vi "rsidr_core_global.vi"() -> ()   [LabVIEW 2015, in "Rohde&Schwarz CMXP NR FR2 Measurement.lvlib"] (continued)
{"Level"=5, "Class Only"=FALSE, "Identifier"="RSCMXPNRFR2M_ATTR_QUERY_MULTI_EVAL_MEASUREMENT_LIST_TERR_EXTREME_LIMIT_CHECK_RESULTS", "Descriptive Name"="Query Multi Eval Measurement List TERR Extreme Limit Check Results", "Data Type"=enum."RawString", "Command"="CALC:NRMM:MEAS{instance}:MEV:LIST:MOD:TERR:EXTR?", "Access"=enum."Read Only", "Range Table"="", "Read Callback"="", "Write Callback"="", "Range Callback"="", "Check Callback"="", "Rngtable Callback"="", "Coerce Callback"="", "Supported Models"="", "Instrument Options"="", "Check Status Callback"="", "Flags"=0, "Help"="Returns the limit check results for the transmit time error values for all measured list mode segments.\n\nAvailable Repeated Capabilities:\ninstance: i0, i1, i2, i3, i4, i5, i6, i7, i8, i9, i10, i11, i12, i13, i14, i15, i16, i17, i18, i19, i20, i21, i22, i23, i24, i25, i26, i27, i28, i29, i30, i31, i32\r\n\nRemote-control command(s):\nCALCulate:NRMMw:MEAS<i>:MEValuation:LIST:MODulation:TERRor:EXTReme?"}, {"Level"=5, "Class Only"=FALSE, "Identifier"="RSCMXPNRFR2M_ATTR_FETCH_MULTI_EVAL_MEASUREMENT_LIST_TERR_STANDARD_DEVIATION_RESULTS", "Descriptive Name"="Fetch Multi Eval Measurement List TERR Standard Deviation Results", "Data Type"=enum."RawString", "Command"="FETC:NRMM:MEAS{instance}:MEV:LIST:MOD:TERR:SDEV?", "Access"=enum."Read Only", "Range Table"="", "Read Callback"="", "Write Callback"="", "Range Callback"="", "Check Callback"="", "Rngtable Callback"="", "Coerce Callback"="", "Supported Models"="", "Instrument Options"="", "Check Status Callback"="", "Flags"=0, "Help"="Returns transmit time error values for all measured list mode segments.\n\nAvailable Repeated Capabilities:\ninstance: i0, i1, i2, i3, i4, i5, i6, i7, i8, i9, i10, i11, i12, i13, i14, i15, i16, i17, i18, i19, i20, i21, i22, i23, i24, i25, i26, i27, i28, i29, i30, i31, i32\r\n\nRemote-control command(s):\nFETCh:NRMMw:MEAS<i>:MEValuation:LIST:MODulation:TERRor:SDEViation?"}, {"Level"=4, "Class Only"=TRUE, "Identifier"="", "Descriptive Name"="User Equipment Power", "Data Type"=enum."ViInt32", "Command"="", "Access"=enum."Read Only", "Range Table"="", "Read Callback"="", "Write Callback"="", "Range Callback"="", "Check Callback"="", "Rngtable Callback"="", "Coerce Callback"="", "Supported Models"="", "Instrument Options"="", "Check Status Callback"="", "Flags"=0, "Help"="The following attributes return user equipment power values for all measured list mode segments."}, {"Level"=5, "Class Only"=FALSE, "Identifier"="RSCMXPNRFR2M_ATTR_FETCH_MULTI_EVAL_MEASUREMENT_LIST_TPOWER_AVERAGE_RESULTS", "Descriptive Name"="Fetch Multi Eval Measurement List TPower Average Results", "Data Type"=enum."RawString", "Command"="FETC:NRMM:MEAS{instance}:MEV:LIST:MOD:TPOW:AVER?", "Access"=enum."Read Only", "Range Table"="", "Read Callback"="", "Write Callback"="", "Range Callback"="", "Check Callback"="", "Rngtable Callback"="", "Coerce Callback"="", "Supported Models"="", "Instrument Options"="", "Check Status Callback"="", "Flags"=0, "Help"="Returns user equipment power values for all measured list mode segments.\n\nAvailable Repeated Capabilities:\ninstance: i0, i1, i2, i3, i4, i5, i6, i7, i8, i9, i10, i11, i12, i13, i14, i15, i16, i17, i18, i19, i20, i21, i22, i23, i24, i25, i26, i27, i28, i29, i30, i31, i32\r\n\nRemote-control command(s):\nFETCh:NRMMw:MEAS<i>:MEValuation:LIST:MODulation:TPOWer:AVERage?"}, {"Level"=5, "Class Only"=FALSE, "Identifier"="RSCMXPNRFR2M_ATTR_FETCH_MULTI_EVAL_MEASUREMENT_LIST_TPOWER_CURRENT_RESULTS", "Descriptive Name"="Fetch Multi Eval Measurement List TPower Current Results", "Data Type"=enum."RawString", "Command"="FETC:NRMM:MEAS{instance}:MEV:LIST:MOD:TPOW:CURR?", "Access"=enum."Read Only", "Range Table"="", "Read Callback"="", "Write Callback"="", "Range Callback"="", "Check Callback"="", "Rngtable Callback"="", "Coerce Callback"="", "Supported Models"="", "Instrument Options"="", "Check Status Callback"="", "Flags"=0, "Help"="Returns user equipment power values for all measured list mode segments.\n\nAvailable Repeated Capabilities:\ninstance: i0, i1, i2, i3, i4, i5, i6, i7, i8, i9, i10, i11, i12, i13, i14, i15, i16, i17, i18, i19, i20, i21, i22, i23, i24, i25, i26, i27, i28, i29, i30, i31, i32\r\n\nRemote-control command(s):\nFETCh:NRMMw:MEAS<i>:MEValuation:LIST:MODulation:TPOWer:CURRent?"}, {"Level"=5, "Class Only"=FALSE, "Identifier"="RSCMXPNRFR2M_ATTR_FETCH_MULTI_EVAL_MEASUREMENT_LIST_TPOWER_MAXIMUM_RESULTS", "Descriptive Name"="Fetch Multi Eval Measurement List TPower Maximum Results", "Data Type"=enum."RawString", "Command"="FETC:NRMM:MEAS{instance}:MEV:LIST:MOD:TPOW:MAX?", "Access"=enum."Read Only", "Range Table"="", "Read Callback"="", "Write Callback"="", "Range Callback"="", "Check Callback"="", "Rngtable Callback"="", "Coerce Callback"="", "Supported Models"="", "Instrument Options"="", "Check Status Callback"="", "Flags"=0, "Help"="Returns user equipment power values for all measured list mode segments.\n\nAvailable Repeated Capabilities:\ninstance: i0, i1, i2, i3, i4, i5, i6, i7, i8, i9, i10, i11, i12, i13, i14, i15, i16, i17, i18, i19, i20, i21, i22, i23, i24, i25, i26, i27, i28, i29, i30, i31, i32\r\n\nRemote-control command(s):\nFETCh:NRMMw:MEAS<i>:MEValuation:LIST:MODulation:TPOWer:MAXimum?"}, {"Level"=5, "Class Only"=FALSE, "Identifier"="RSCMXPNRFR2M_ATTR_FETCH_MULTI_EVAL_MEASUREMENT_LIST_TPOWER_MINIMUM_RESULTS", "Descriptive Name"="Fetch Multi Eval Measurement List TPower Minimum Results", "Data Type"=enum."RawString", "Command"="FETC:NRMM:MEAS{instance}:MEV:LIST:MOD:TPOW:MIN?", "Access"=enum."Read Only", "Range Table"="", "Read Callback"="", "Write Callback"="", "Range Callback"="", "Check Callback"="", "Rngtable Callback"="", "Coerce Callback"="", "Supported Models"="", "Instrument Options"="", "Check Status Callback"="", "Flags"=0, "Help"="Returns user equipment power values for all measured list mode segments.\n\nAvailable Repeated Capabilities:\ninstance: i0, i1, i2, i3, i4, i5, i6, i7, i8, i9, i10, i11, i12, i13, i14, i15, i16, i17, i18, i19, i20, i21, i22, i23, i24, i25, i26, i27, i28, i29, i30, i31, i32\r\n\nRemote-control command(s):\nFETCh:NRMMw:MEAS<i>:MEValuation:LIST:MODulation:TPOWer:MINimum?"}, {"Level"=5, "Class Only"=FALSE, "Identifier"="RSCMXPNRFR2M_ATTR_FETCH_MULTI_EVAL_MEASUREMENT_LIST_TPOWER_STANDARD_DEVIATION_RESULTS", "Descriptive Name"="Fetch Multi Eval Measurement List TPower Standard Deviation Results", "Data Type"=enum."RawString", "Command"="FETC:NRMM:MEAS{instance}:MEV:LIST:MOD:TPOW:SDEV?", "Access"=enum."Read Only", "Range Table"="", "Read Callback"="", "Write Callback"="", "Range Callback"="", "Check Callback"="", "Rngtable Callback"="", "Coerce Callback"="", "Supported Models"="", "Instrument Options"="", "Check Status Callback"="", "Flags"=0, "Help"="Returns user equipment power values for all measured list mode segments.\n\nAvailable Repeated Capabilities:\ninstance: i0, i1, i2, i3, i4, i5, i6, i7, i8, i9, i10, i11, i12, i13, i14, i15, i16, i17, i18, i19, i20, i21, i22, i23, i24, i25, i26, i27, i28, i29, i30, i31, i32\r\n\nRemote-control command(s):\nFETCh:NRMMw:MEAS<i>:MEValuation:LIST:MODulation:TPOWer:SDEViation?"}, {"Level"=5, "Class Only"=FALSE, "Identifier"="RSCMXPNRFR2M_ATTR_QUERY_MULTI_EVAL_MEASUREMENT_LIST_TPOWER_AVERAGE_LIMIT_CHECK_RESULTS", "Descriptive Name"="Query Multi Eval Measurement List TPower Average Limit Check Results", "Data Type"=enum."RawString", "Command"="CALC:NRMM:MEAS{instance}:MEV:LIST:MOD:TPOW:AVER?", "Access"=enum."Read Only", "Range Table"="", "Read Callback"="", "Write Callback"="", "Range Callback"="", "Check Callback"="", "Rngtable Callback"="", "Coerce Callback"="", "Supported Models"="", "Instrument Options"="", "Check Status Callback"="", "Flags"=0, "Help"="Returns the limit check results for the user equipment power values for all measured list mode segments.\n\nAvailable Repeated Capabilities:\ninstance: i0, i1, i2, i3, i4, i5, i6, i7, i8, i9, i10, i11, i12, i13, i14, i15, i16, i17, i18, i19, i20, i21, i22, i23, i24, i25, i26, i27, i28, i29, i30, i31, i32\r\n\nRemote-control command(s):\nCALCulate:NRMMw:MEAS<i>:MEValuation:LIST:MODulation:TPOWer:AVERage?"}, {"Level"=5, "Class Only"=FALSE, "Identifier"="RSCMXPNRFR2M_ATTR_QUERY_MULTI_EVAL_MEASUREMENT_LIST_TPOWER_CURRENT_LIMIT_CHECK_RESULTS", "Descriptive Name"="Query Multi Eval Measurement List TPower Current Limit Check Results", "Data Type"=enum."RawString", "Command"="CALC:NRMM:MEAS{instance}:MEV:LIST:MOD:TPOW:CURR?", "Access"=enum."Read Only", "Range Table"="", "Read Callback"="", "Write Callback"="", "Range Callback"="", "Check Callback"="", "Rngtable Callback"="", "Coerce Callback"="", "Supported Models"="", "Instrument Options"="", "Check Status Callback"="", "Flags"=0, "Help"="Returns the limit check results for the user equipment power values for all measured list mode segments.\n\nAvailable Repeated Capabilities:\ninstance: i0, i1, i2, i3, i4, i5, i6, i7, i8, i9, i10, i11, i12, i13, i14, i15, i16, i17, i18, i19, i20, i21, i22, i23, i24, i25, i26, i27, i28, i29, i30, i31, i32\r\n\nRemote-control command(s):\nCALCulate:NRMMw:MEAS<i>:MEValuation:LIST:MODulation:TPOWer:CURRent?"}, {"Level"=5, "Class Only"=FALSE, "Identifier"="RSCMXPNRFR2M_ATTR_QUERY_MULTI_EVAL_MEASUREMENT_LIST_TPOWER_MAXIMUM_LIMIT_CHECK_RESULTS", "Descriptive Name"="Query Multi Eval Measurement List TPower Maximum Limit Check Results", "Data Type"=enum."RawString", "Command"="CALC:NRMM:MEAS{instance}:MEV:LIST:MOD:TPOW:MAX?", "Access"=enum."Read Only", "Range Table"="", "Read Callback"="", "Write Callback"="", "Range Callback"="", "Check Callback"="", "Rngtable Callback"="", "Coerce Callback"="", "Supported Models"="", "Instrument Options"="", "Check Status Callback"="", "Flags"=0, "Help"="Returns the limit check results for the user equipment power values for all measured list mode segments.\n\nAvailable Repeated Capabilities:\ninstance: i0, i1, i2, i3, i4, i5, i6, i7, i8, i9, i10, i11, i12, i13, i14, i15, i16, i17, i18, i19, i20, i21, i22, i23, i24, i25, i26, i27, i28, i29, i30, i31, i32\r\n\nRemote-control command(s):\nCALCulate:NRMMw:MEAS<i>:MEValuation:LIST:MODulation:TPOWer:MAXimum?"}, {"Level"=5, "Class Only"=FALSE, "Identifier"="RSCMXPNRFR2M_ATTR_QUERY_MULTI_EVAL_MEASUREMENT_LIST_TPOWER_MINIMUM_LIMIT_CHECK_RESULTS", "Descriptive Name"="Query Multi Eval Measurement List TPower Minimum Limit Check Results", "Data Type"=enum."RawString", "Command"="CALC:NRMM:MEAS{instance}:MEV:LIST:MOD:TPOW:MIN?", "Access"=enum."Read Only", "Range Table"="", "Read Callback"="", "Write Callback"="", "Range Callback"="", "Check Callback"="", "Rngtable Callback"="", "Coerce Callback"="", "Supported Models"="", "Instrument Options"="", "Check Status Callback"="", "Flags"=0, "Help"="Returns the limit check results for the user equipment power values for all measured list mode segments.\n\nAvailable Repeated Capabilities:\ninstance: i0, i1, i2, i3, i4, i5, i6, i7, i8, i9, i10, i11, i12, i13, i14, i15, i16, i17, i18, i19, i20, i21, i22, i23, i24, i25, i26, i27, i28, i29, i30, i31, i32\r\n\nRemote-control command(s):\nCALCulate:NRMMw:MEAS<i>:MEValuation:LIST:MODulation:TPOWer:MINimum?"}, {"Level"=4, "Class Only"=TRUE, "Identifier"="", "Descriptive Name"="Modulation", "Data Type"=enum."ViInt32", "Command"="", "Access"=enum."Read Only", "Range Table"="", "Read Callback"="", "Write Callback"="", "Range Callback"="", "Check Callback"="", "Rngtable Callback"="", "Coerce Callback"="", "Supported Models"="", "Instrument Options"="", "Check Status Callback"="", "Flags"=0, "Help"="The following attributes return the detected modulation scheme for all measured list mode segments."}, {"Level"=5, "Class Only"=FALSE, "Identifier"="RSCMXPNRFR2M_ATTR_FETCH_MULTI_EVAL_MEASUREMENT_LIST_MODULATION_DETECTED_ALLOCATION_RESULTS", "Descriptive Name"="Fetch Multi Eval Measurement List Modulation Detected Allocation Results", "Data Type"=enum."RawString", "Command"="FETC:NRMM:MEAS{instance}:MEV:LIST:MOD:DALL?", "Access"=enum."Read Only", "Range Table"="", "Read Callback"="", "Write Callback"="", "Range Callback"="", "Check Callback"="", "Rngtable Callback"="", "Coerce Callback"="", "Supported Models"="", "Instrument Options"="", "Check Status Callback"="", "Flags"=0, "Help"="Returns the detected allocation for all measured list mode segments.\n\nAvailable Repeated Capabilities:\ninstance: i0, i1, i2, i3, i4, i5, i6, i7, i8, i9, i10, i11, i12, i13, i14, i15, i16, i17, i18, i19, i20, i21, i22, i23, i24, i25, i26, i27, i28, i29, i30, i31, i32\r\n\nRemote-control command(s):\nFETCh:NRMMw:MEAS<i>:MEValuation:LIST:MODulation:DALLocation?"}, {"Level"=5, "Class Only"=FALSE, "Identifier"="RSCMXPNRFR2M_ATTR_FETCH_MULTI_EVAL_MEASUREMENT_LIST_MODULATION_DETECTED_MODULATION_RESULTS", "Descriptive Name"="Fetch Multi Eval Measurement List Modulation Detected Modulation Results", "Data Type"=enum."RawString", "Command"="FETC:NRMM:MEAS{instance}:MEV:LIST:MOD:DMOD?", "Access"=enum."Read Only", "Range Table"="", "Read Callback"="", "Write Callback"="", "Range Callback"="", "Check Callback"="", "Rngtable Callback"="", "Coerce Callback"="", "Supported Models"="", "Instrument Options"="", "Check Status Callback"="", "Flags"=0, "Help"="Returns the detected modulation scheme for all measured list mode segments.\n\nAvailable Repeated Capabilities:\ninstance: i0, i1, i2, i3, i4, i5, i6, i7, i8, i9, i10, i11, i12, i13, i14, i15, i16, i17, i18, i19, i20, i21, i22, i23, i24, i25, i26, i27, i28, i29, i30, i31, i32\r\n\nRemote-control command(s):\nFETCh:NRMMw:MEAS<i>:MEValuation:LIST:MODulation:DMODulation?"}, {"Level"=4, "Class Only"=TRUE, "Identifier"="", "Descriptive Name"="Spectrum Emission Mask", "Data Type"=enum."ViInt32", "Command"="", "Access"=enum."Read Only", "Range Table"="", "Read Callback"="", "Write Callback"="", "Range Callback"="", "Check Callback"="", "Rngtable Callback"="", "Coerce Callback"="", "Supported Models"="", "Instrument Options"="", "Check Status Callback"="", "Flags"=0, "Help"="The following attributes return the occupied bandwidth for all measured list mode segments."}, {"Level"=5, "Class Only"=FALSE, "Identifier"="RSCMXPNRFR2M_ATTR_FETCH_MULTI_EVAL_MEASUREMENT_LIST_SEM_OBW_AVERAGE_RESULTS", "Descriptive Name"="Fetch Multi Eval Measurement List SEM OBW Average Results", "Data Type"=enum."RawString", "Command"="FETC:NRMM:MEAS{instance}:MEV:LIST:SEM:OBW:AVER?", "Access"=enum."Read Only", "Range Table"="", "Read Callback"="", "Write Callback"="", "Range Callback"="", "Check Callback"="", "Rngtable Callback"="", "Coerce Callback"="", "Supported Models"="", "Instrument Options"="", "Check Status Callback"="", "Flags"=0, "Help"="Returns the occupied bandwidth for all measured list mode segments.\n\nAvailable Repeated Capabilities:\ninstance: i0, i1, i2, i3, i4, i5, i6, i7, i8, i9, i10, i11, i12, i13, i14, i15, i16, i17, i18, i19, i20, i21, i22, i23, i24, i25, i26, i27, i28, i29, i30, i31, i32\r\n\nRemote-control command(s):\nFETCh:NRMMw:MEAS<i>:MEValuation:LIST:SEMask:OBW:AVERage?"}, {"Level"=5, "Class Only"=FALSE, "Identifier"="RSCMXPNRFR2M_ATTR_FETCH_MULTI_EVAL_MEASUREMENT_LIST_SEM_OBW_CURRENT_RESULTS", "Descriptive Name"="Fetch Multi Eval Measurement List SEM OBW Current Results", "Data Type"=enum."RawString", "Command"="FETC:NRMM:MEAS{instance}:MEV:LIST:SEM:OBW:CURR?", "Access"=enum."Read Only", "Range Table"="", "Read Callback"="", "Write Callback"="", "Range Callback"="", "Check Callback"="", "Rngtable Callback"="", "Coerce Callback"="", "Supported Models"="", "Instrument Options"="", "Check Status Callback"="", "Flags"=0, "Help"="Returns the occupied bandwidth for all measured list mode segments.\n\nAvailable Repeated Capabilities:\ninstance: i0, i1, i2, i3, i4, i5, i6, i7, i8, i9, i10, i11, i12, i13, i14, i15, i16, i17, i18, i19, i20, i21, i22, i23, i24, i25, i26, i27, i28, i29, i30, i31, i32\r\n\nRemote-control command(s):\nFETCh:NRMMw:MEAS<i>:MEValuation:LIST:SEMask:OBW:CURRent?"}, {"Level"=5, "Class Only"=FALSE, "Identifier"="RSCMXPNRFR2M_ATTR_FETCH_MULTI_EVAL_MEASUREMENT_LIST_SEM_OBW_EXTREME_RESULTS", "Descriptive Name"="Fetch Multi Eval Measurement List SEM OBW Extreme Results", "Data Type"=enum."RawString", "Command"="FETC:NRMM:MEAS{instance}:MEV:LIST:SEM:OBW:EXTR?", "Access"=enum."Read Only", "Range Table"="", "Read Callback"="", "Write Callback"="", "Range Callback"="", "Check Callback"="", "Rngtable Callback"="", "Coerce Callback"="", "Supported Models"="", "Instrument Options"="", "Check Status Callback"="", "Flags"=0, "Help"="Returns the occupied bandwidth for all measured list mode segments.\n\nAvailable Repeated Capabilities:\ninstance: i0, i1, i2, i3, i4, i5, i6, i7, i8, i9, i10, i11, i12, i13, i14, i15, i16, i17, i18, i19, i20, i21, i22, i23, i24, i25, i26, i27, i28, i29, i30, i31, i32\r\n\nRemote-control command(s):\nFETCh:NRMMw:MEAS<i>:MEValuation:LIST:SEMask:OBW:EXTReme?"}, {"Level"=5, "Class Only"=FALSE, "Identifier"="RSCMXPNRFR2M_ATTR_FETCH_MULTI_EVAL_MEASUREMENT_LIST_SEM_OBW_STANDARD_DEVIATION_RESULTS", "Descriptive Name"="Fetch Multi Eval Measurement List SEM OBW Standard Deviation Results", "Data Type"=enum."RawString", "Command"="FETC:NRMM:MEAS{instance}:MEV:LIST:SEM:OBW:SDEV?", "Access"=enum."Read Only", "Range Table"="", "Read Callback"="", "Write Callback"="", "Range Callback"="", "Check Callback"="", "Rngtable Callback"="", "Coerce Callback"="", "Supported Models"="", "Instrument Options"="", "Check Status Callback"="", "Flags"=0, "Help"="Returns the occupied bandwidth for all measured list mode segments.\n\nAvailable Repeated Capabilities:\ninstance: i0, i1, i2, i3, i4, i5, i6, i7, i8, i9, i10, i11, i12, i13, i14, i15, i16, i17, i18, i19, i20, i21, i22, i23, i24, i25, i26, i27, i28, i29, i30, i31, i32\r\n\nRemote-control command(s):\nFETCh:NRMMw:MEAS<i>:MEValuation:LIST:SEMask:OBW:SDEViation?"}, {"Level"=5, "Class Only"=FALSE, "Identifier"="RSCMXPNRFR2M_ATTR_QUERY_MULTI_EVAL_MEASUREMENT_LIST_SEM_OBW_AVERAGE_LIMIT_CHECK_RESULTS", "Descriptive Name"="Query Multi Eval Measurement List SEM OBW Average Limit Check Results", "Data Type"=enum."RawString", "Command"="CALC:NRMM:MEAS{instance}:MEV:LIST:SEM:OBW:AVER?", "Access"=enum."Read Only", "Range Table"="", "Read Callback"="", "Write Callback"="", "Range Callback"="", "Check Callback"="", "Rngtable Callback"="", "Coerce Callback"="", "Supported Models"="", "Instrument Options"="", "Check Status Callback"="", "Flags"=0, "Help"="Returns the limit check results for the occupied bandwidth for all measured list mode segments.\n\nAvailable Repeated Capabilities:\ninstance: i0, i1, i2, i3, i4, i5, i6, i7, i8, i9, i10, i11, i12, i13, i14, i15, i16, i17, i18, i19, i20, i21, i22, i23, i24, i25, i26, i27, i28, i29, i30, i31, i32\r\n\nRemote-control command(s):\nCALCulate:NRMMw:MEAS<i>:MEValuation:LIST:SEMask:OBW:AVERage?"}, {"Level"=5, "Class Only"=FALSE, "Identifier"="RSCMXPNRFR2M_ATTR_QUERY_MULTI_EVAL_MEASUREMENT_LIST_SEM_OBW_CURRENT_LIMIT_CHECK_RESULTS", "Descriptive Name"="Query Multi Eval Measurement List SEM OBW Current Limit Check Results", "Data Type"=enum."RawString", "Command"="CALC:NRMM:MEAS{instance}:MEV:LIST:SEM:OBW:CURR?", "Access"=enum."Read Only", "Range Table"="", "Read Callback"="", "Write Callback"="", "Range Callback"="", "Check Callback"="", "Rngtable Callback"="", "Coerce Callback"="", "Supported Models"="", "Instrument Options"="", "Check Status Callback"="", "Flags"=0, "Help"="Returns the limit check results for the occupied bandwidth for all measured list mode segments.\n\nAvailable Repeated Capabilities:\ninstance: i0, i1, i2, i3, i4, i5, i6, i7, i8, i9, i10, i11, i12, i13, i14, i15, i16, i17, i18, i19, i20, i21, i22, i23, i24, i25, i26, i27, i28, i29, i30, i31, i32\r\n\nRemote-control command(s):\nCALCulate:NRMMw:MEAS<i>:MEValuation:LIST:SEMask:OBW:CURRent?"}, {"Level"=5, "Class Only"=FALSE, "Identifier"="RSCMXPNRFR2M_ATTR_QUERY_MULTI_EVAL_MEASUREMENT_LIST_SEM_OBW_EXTREME_LIMIT_CHECK_RESULTS", "Descriptive Name"="Query Multi Eval Measurement List SEM OBW Extreme Limit Check Results", "Data Type"=enum."RawString", "Command"="CALC:NRMM:MEAS{instance}:MEV:LIST:SEM:OBW:EXTR?", "Access"=enum."Read Only", "Range Table"="", "Read Callback"="", "Write Callback"="", "Range Callback"="", "Check Callback"="", "Rngtable Callback"="", "Coerce Callback"="", "Supported Models"="", "Instrument Options"="", "Check Status Callback"="", "Flags"=0, "Help"="Returns the limit check results for the occupied bandwidth for all measured list mode segments.\n\nAvailable Repeated Capabilities:\ninstance: i0, i1, i2, i3, i4, i5, i6, i7, i8, i9, i10, i11, i12, i13, i14, i15, i16, i17, i18, i19, i20, i21, i22, i23, i24, i25, i26, i27, i28, i29, i30, i31, i32\r\n\nRemote-control command(s):\nCALCulate:NRMMw:MEAS<i>:MEValuation:LIST:SEMask:OBW:EXTReme?"}, {"Level"=5, "Class Only"=FALSE, "Identifier"="RSCMXPNRFR2M_ATTR_FETCH_MULTI_EVAL_MEASUREMENT_LIST_SEM_TX_POWER_AVERAGE_RESULTS", "Descriptive Name"="Fetch Multi Eval Measurement List SEM TX Power Average Results", "Data Type"=enum."RawString", "Command"="FETC:NRMM:MEAS{instance}:MEV:LIST:SEM:TXP:AVER?", "Access"=enum."Read Only", "Range Table"="", "Read Callback"="", "Write Callback"="", "Range Callback"="", "Check Callback"="", "Rngtable Callback"="", "Coerce Callback"="", "Supported Models"="", "Instrument Options"="", "Check Status Callback"="", "Flags"=0, "Help"="Returns the total TX power in the slot for all measured list mode segments.\n\nAvailable Repeated Capabilities:\ninstance: i0, i1, i2, i3, i4, i5, i6, i7, i8, i9, i10, i11, i12, i13, i14, i15, i16, i17, i18, i19, i20, i21, i22, i23, i24, i25, i26, i27, i28, i29, i30, i31, i32\r\n\nRemote-control command(s):\nFETCh:NRMMw:MEAS<i>:MEValuation:LIST:SEMask:TXPower:AVERage?"}, {"Level"=5, "Class Only"=FALSE, "Identifier"="RSCMXPNRFR2M_ATTR_FETCH_MULTI_EVAL_MEASUREMENT_LIST_SEM_TX_POWER_CURRENT_RESULTS", "Descriptive Name"="Fetch Multi Eval Measurement List SEM TX Power Current Results", "Data Type"=enum."RawString", "Command"="FETC:NRMM:MEAS{instance}:MEV:LIST:SEM:TXP:CURR?", "Access"=enum."Read Only", "Range Table"="", "Read Callback"="", "Write Callback"="", "Range Callback"="", "Check Callback"="", "Rngtable Callback"="", "Coerce Callback"="", "Supported Models"="", "Instrument Options"="", "Check Status Callback"="", "Flags"=0, "Help"="Returns the total TX power in the slot for all measured list mode segments.\n\nAvailable Repeated Capabilities:\ninstance: i0, i1, i2, i3, i4, i5, i6, i7, i8, i9, i10, i11, i12, i13, i14, i15, i16, i17, i18, i19, i20, i21, i22, i23, i24, i25, i26, i27, i28, i29, i30, i31, i32\r\n\nRemote-control command(s):\nFETCh:NRMMw:MEAS<i>:MEValuation:LIST:SEMask:TXPower:CURRent?"}, {"Level"=5, "Class Only"=FALSE, "Identifier"="RSCMXPNRFR2M_ATTR_FETCH_MULTI_EVAL_MEASUREMENT_LIST_SEM_TX_POWER_STANDARD_DEVIATION_RESULTS", "Descriptive Name"="Fetch Multi Eval Measurement List SEM TX Power Standard Deviation Results", "Data Type"=enum."RawString", "Command"="FETC:NRMM:MEAS{instance}:MEV:LIST:SEM:TXP:SDEV?", "Access"=enum."Read Only", "Range Table"="", "Read Callback"="", "Write Callback"="", "Range Callback"="", "Check Callback"="", "Rngtable Callback"="", "Coerce Callback"="", "Supported Models"="", "Instrument Options"="", "Check Status Callback"="", "Flags"=0, "Help"="Returns the total TX power in the slot for all measured list mode segments.\n\nAvailable Repeated Capabilities:\ninstance: i0, i1, i2, i3, i4, i5, i6, i7, i8, i9, i10, i11, i12, i13, i14, i15, i16, i17, i18, i19, i20, i21, i22, i23, i24, i25, i26, i27, i28, i29, i30, i31, i32\r\n\nRemote-control command(s):\nFETCh:NRMMw:MEAS<i>:MEValuation:LIST:SEMask:TXPower:SDEViation?"}, {"Level"=5, "Class Only"=FALSE, "Identifier"="RSCMXPNRFR2M_ATTR_FETCH_MULTI_EVAL_MEASUREMENT_LIST_SEM_TX_POWER_MAXIMUM_RESULTS", "Descriptive Name"="Fetch Multi Eval Measurement List SEM TX Power Maximum Results", "Data Type"=enum."RawString", "Command"="FETC:NRMM:MEAS{instance}:MEV:LIST:SEM:TXP:MAX?", "Access"=enum."Read Only", "Range Table"="", "Read Callback"="", "Write Callback"="", "Range Callback"="", "Check Callback"="", "Rngtable Callback"="", "Coerce Callback"="", "Supported Models"="", "Instrument Options"="", "Check Status Callback"="", "Flags"=0, "Help"="Returns the total TX power in the slot for all measured list mode segments.\n\nAvailable Repeated Capabilities:\ninstance: i0, i1, i2, i3, i4, i5, i6, i7, i8, i9, i10, i11, i12, i13, i14, i15, i16, i17, i18, i19, i20, i21, i22, i23, i24, i25, i26, i27, i28, i29, i30, i31, i32\r\n\nRemote-control command(s):\nFETCh:NRMMw:MEAS<i>:MEValuation:LIST:SEMask:TXPower:MAXimum?"}, {"Level"=5, "Class Only"=FALSE, "Identifier"="RSCMXPNRFR2M_ATTR_FETCH_MULTI_EVAL_MEASUREMENT_LIST_SEM_TX_POWER_MINIMUM_RESULTS", "Descriptive Name"="Fetch Multi Eval Measurement List SEM TX Power Minimum Results", "Data Type"=enum."RawString", "Command"="FETC:NRMM:MEAS{instance}:MEV:LIST:SEM:TXP:MIN?", "Access"=enum."Read Only", "Range Table"="", "Read Callback"="", "Write Callback"="", "Range Callback"="", "Check Callback"="", "Rngtable Callback"="", "Coerce Callback"="", "Supported Models"="", "Instrument Options"="", "Check Status Callback"="", "Flags"=0, "Help"="Returns the total TX power in the slot for all measured list mode segments.\n\nAvailable Repeated Capabilities:\ninstance: i0, i1, i2, i3, i4, i5, i6, i7, i8, i9, i10, i11, i12, i13, i14, i15, i16, i17, i18, i19, i20, i21, i22, i23, i24, i25, i26, i27, i28, i29, i30, i31, i32\r\n\nRemote-control command(s):\nFETCh:NRMMw:MEAS<i>:MEValuation:LIST:SEMask:TXPower:MINimum?"}, {"Level"=5, "Class Only"=FALSE, "Identifier"="RSCMXPNRFR2M_ATTR_QUERY_MULTI_EVAL_MEASUREMENT_LIST_SEM_TX_POWER_AVERAGE_LIMIT_CHECK_RESULTS", "Descriptive Name"="Query Multi Eval Measurement List SEM TX Power Average Limit Check Results", "Data Type"=enum."RawString", "Command"="CALC:NRMM:MEAS{instance}:MEV:LIST:SEM:TXP:AVER?", "Access"=enum."Read Only", "Range Table"="", "Read Callback"="", "Write Callback"="", "Range Callback"="", "Check Callback"="", "Rngtable Callback"="", "Coerce Callback"="", "Supported Models"="", "Instrument Options"="", "Check Status Callback"="", "Flags"=0, "Help"="Returns the limit check results for the total TX power in the slot for all measured list mode segments.\n\nAvailable Repeated Capabilities:\ninstance: i0, i1, i2, i3, i4, i5, i6, i7, i8, i9, i10, i11, i12, i13, i14, i15, i16, i17, i18, i19, i20, i21, i22, i23, i24, i25, i26, i27, i28, i29, i30, i31, i32\r\n\nRemote-control command(s):\nCALCulate:NRMMw:MEAS<i>:MEValuation:LIST:SEMask:TXPower:AVERage?"}, {"Level"=5, "Class Only"=FALSE, "Identifier"="RSCMXPNRFR2M_ATTR_QUERY_MULTI_EVAL_MEASUREMENT_LIST_SEM_TX_POWER_CURRENT_LIMIT_CHECK_RESULTS", "Descriptive Name"="Query Multi Eval Measurement List SEM TX Power Current Limit Check Results", "Data Type"=enum."RawString", "Command"="CALC:NRMM:MEAS{instance}:MEV:LIST:SEM:TXP:CURR?", "Access"=enum."Read Only", "Range Table"="", "Read Callback"="", "Write Callback"="", "Range Callback"="", "Check Callback"="", "Rngtable Callback"="", "Coerce Callback"="", "Supported Models"="", "Instrument Options"="", "Check Status Callback"="", "Flags"=0, "Help"="Returns the limit check results for the total TX power in the slot for all measured list mode segments.\n\nAvailable Repeated Capabilities:\ninstance: i0, i1, i2, i3, i4, i5, i6, i7, i8, i9, i10, i11, i12, i13, i14, i15, i16, i17, i18, i19, i20, i21, i22, i23, i24, i25, i26, i27, i28, i29, i30, i31, i32\r\n\nRemote-control command(s):\nCALCulate:NRMMw:MEAS<i>:MEValuation:LIST:SEMask:TXPower:CURRent?"}, {"Level"=5, "Class Only"=FALSE, "Identifier"="RSCMXPNRFR2M_ATTR_QUERY_MULTI_EVAL_MEASUREMENT_LIST_SEM_TX_POWER_MAXIMUM_LIMIT_CHECK_RESULTS", "Descriptive Name"="Query Multi Eval Measurement List SEM TX Power Maximum Limit Check Results", "Data Type"=enum."RawString", "Command"="CALC:NRMM:MEAS{instance}:MEV:LIST:SEM:TXP:MAX?", "Access"=enum."Read Only", "Range Table"="", "Read Callback"="", "Write Callback"="", "Range Callback"="", "Check Callback"="", "Rngtable Callback"="", "Coerce Callback"="", "Supported Models"="", "Instrument Options"="", "Check Status Callback"="", "Flags"=0, "Help"="Returns the limit check results for the total TX power in the slot for all measured list mode segments.\n\nAvailable Repeated Capabilities:\ninstance: i0, i1, i2, i3, i4, i5, i6, i7, i8, i9, i10, i11, i12, i13, i14, i15, i16, i17, i18, i19, i20, i21, i22, i23, i24, i25, i26, i27, i28, i29, i30, i31, i32\r\n\nRemote-control command(s):\nCALCulate:NRMMw:MEAS<i>:MEValuation:LIST:SEMask:TXPower:MAXimum?"}, {"Level"=5, "Class Only"=FALSE, "Identifier"="RSCMXPNRFR2M_ATTR_QUERY_MULTI_EVAL_MEASUREMENT_LIST_SEM_TX_POWER_MINIMUM_LIMIT_CHECK_RESULTS", "Descriptive Name"="Query Multi Eval Measurement List SEM TX Power Minimum Limit Check Results", "Data Type"=enum."RawString", "Command"="CALC:NRMM:MEAS{instance}:MEV:LIST:SEM:TXP:MIN?", "Access"=enum."Read Only", "Range Table"="", "Read Callback"="", "Write Callback"="", "Range Callback"="", "Check Callback"="", "Rngtable Callback"="", "Coerce Callback"="", "Supported Models"="", "Instrument Options"="", "Check Status Callback"="", "Flags"=0, "Help"="Returns the limit check results for the total TX power in the slot for all measured list mode segments.\n\nAvailable Repeated Capabilities:\ninstance: i0, i1, i2, i3, i4, i5, i6, i7, i8, i9, i10, i11, i12, i13, i14, i15, i16, i17, i18, i19, i20, i21, i22, i23, i24, i25, i26, i27, i28, i29, i30, i31, i32\r\n\nRemote-control command(s):\nCALCulate:NRMMw:MEAS<i>:MEValuation:LIST:SEMask:TXPower:MINimum?"}, {"Level"=5, "Class Only"=FALSE, "Identifier"="RSCMXPNRFR2M_ATTR_FETCH_MULTI_EVAL_MEASUREMENT_LIST_SEM_DETECTED_ALLOCATION_RESULTS", "Descriptive Name"="Fetch Multi Eval Measurement List SEM Detected Allocation Results", "Data Type"=enum."RawString", "Command"="FETC:NRMM:MEAS{instance}:MEV:LIST:SEM:DALL?", "Access"=enum."Read Only", "Range Table"="", "Read Callback"="", "Write Callback"="", "Range Callback"="", "Check Callback"="", "Rngtable Callback"="", "Coerce Callback"="", "Supported Models"="", "Instrument Options"="", "Check Status Callback"="", "Flags"=0, "Help"="Returns the detected allocation for all measured list mode segments.\n\nAvailable Repeated Capabilities:\ninstance: i0, i1, i2, i3, i4, i5, i6, i7, i8, i9, i10, i11, i12, i13, i14, i15, i16, i17, i18, i19, i20, i21, i22, i23, i24, i25, i26, i27, i28, i29, i30, i31, i32\r\n\nRemote-control command(s):\nFETCh:NRMMw:MEAS<i>:MEValuation:LIST:SEMask:DALLocation?"}, {"Level"=5, "Class Only"=TRUE, "Identifier"="", "Descriptive Name"="Area", "Data Type"=enum."ViInt32", "Command"="", "Access"=enum."Read Only", "Range Table"="", "Read Callback"="", "Write Callback"="", "Range Callback"="", "Check Callback"="", "Rngtable Callback"="", "Coerce Callback"="", "Supported Models"="", "Instrument Options"="", "Check Status Callback"="", "Flags"=0, "Help"="The following attributes return spectrum emission mask margin positions for all measured list mode segments."}, {"Level"=6, "Class Only"=FALSE, "Identifier"="RSCMXPNRFR2M_ATTR_FETCH_MULTI_EVAL_MEASUREMENT_LIST_SEM_MARGIN_AREA_NEGATIVE_AVERAGE_RESULTS", "Descriptive Name"="Fetch Multi Eval Measurement List SEM Margin Area Negative Average Results", "Data Type"=enum."RawString", "Command"="FETC:NRMM:MEAS{instance}:MEV:LIST:SEM:MARG:AREA{Area}:NEG:AVER?", "Access"=enum."Read Only", "Range Table"="", "Read Callback"="", "Write Callback"="", "Range Callback"="", "Check Callback"="", "Rngtable Callback"="", "Coerce Callback"="", "Supported Models"="", "Instrument Options"="", "Check Status Callback"="", "Flags"=0, "Help"="Returns spectrum emission mask margin positions for all measured list mode segments.\n\nAvailable Repeated Capabilities:\ninstance: i0, i1, i2, i3, i4, i5, i6, i7, i8, i9, i10, i11, i12, i13, i14, i15, i16, i17, i18, i19, i20, i21, i22, i23, i24, i25, i26, i27, i28, i29, i30, i31, i32\r\nArea: a1, a2, a3, a4, a5, a6, a7, a8, a9, a10, a11, a12\r\n\nRemote-control command(s):\nFETCh:NRMMw:MEAS<i>:MEValuation:LIST:SEMask:MARGin:AREA<no>:NEGativ:AVERage?"}, {"Level"=6, "Class Only"=FALSE, "Identifier"="RSCMXPNRFR2M_ATTR_FETCH_MULTI_EVAL_MEASUREMENT_LIST_SEM_MARGIN_AREA_NEGATIVE_CURRENT_RESULTS", "Descriptive Name"="Fetch Multi Eval Measurement List SEM Margin Area Negative Current Results", "Data Type"=enum."RawString", "Command"="FETC:NRMM:MEAS{instance}:MEV:LIST:SEM:MARG:AREA{Area}:NEG:CURR?", "Access"=enum."Read Only", "Range Table"="", "Read Callback"="", "Write Callback"="", "Range Callback"="", "Check Callback"="", "Rngtable Callback"="", "Coerce Callback"="", "Supported Models"="", "Instrument Options"="", "Check Status Callback"="", "Flags"=0, "Help"="Returns spectrum emission mask margin positions for all measured list mode segments.\n\nAvailable Repeated Capabilities:\ninstance: i0, i1, i2, i3, i4, i5, i6, i7, i8, i9, i10, i11, i12, i13, i14, i15, i16, i17, i18, i19, i20, i21, i22, i23, i24, i25, i26, i27, i28, i29, i30, i31, i32\r\nArea: a1, a2, a3, a4, a5, a6, a7, a8, a9, a10, a11, a12\r\n\nRemote-control command(s):\nFETCh:NRMMw:MEAS<i>:MEValuation:LIST:SEMask:MARGin:AREA<no>:NEGativ:CURRent?"}, {"Level"=6, "Class Only"=FALSE, "Identifier"="RSCMXPNRFR2M_ATTR_FETCH_MULTI_EVAL_MEASUREMENT_LIST_SEM_MARGIN_AREA_NEGATIVE_MINIMUM_RESULTS", "Descriptive Name"="Fetch Multi Eval Measurement List SEM Margin Area Negative Minimum Results", "Data Type"=enum."RawString", "Command"="FETC:NRMM:MEAS{instance}:MEV:LIST:SEM:MARG:AREA{Area}:NEG:MIN?", "Access"=enum."Read Only", "Range Table"="", "Read Callback"="", "Write Callback"="", "Range Callback"="", "Check Callback"="", "Rngtable Callback"="", "Coerce Callback"="", "Supported Models"="", "Instrument Options"="", "Check Status Callback"="", "Flags"=0, "Help"="Returns spectrum emission mask margin positions for all measured list mode segments.\n\nAvailable Repeated Capabilities:\ninstance: i0, i1, i2, i3, i4, i5, i6, i7, i8, i9, i10, i11, i12, i13, i14, i15, i16, i17, i18, i19, i20, i21, i22, i23, i24, i25, i26, i27, i28, i29, i30, i31, i32\r\nArea: a1, a2, a3, a4, a5, a6, a7, a8, a9, a10, a11, a12\r\n\nRemote-control command(s):\nFETCh:NRMMw:MEAS<i>:MEValuation:LIST:SEMask:MARGin:AREA<no>:NEGativ:MINimum?"}, {"Level"=6, "Class Only"=FALSE, "Identifier"="RSCMXPNRFR2M_ATTR_FETCH_MULTI_EVAL_MEASUREMENT_LIST_SEM_MARGIN_AREA_POSITIVE_AVERAGE_RESULTS", "Descriptive Name"="Fetch Multi Eval Measurement List SEM Margin Area Positive Average Results", "Data Type"=enum."RawString", "Command"="FETC:NRMM:MEAS{instance}:MEV:LIST:SEM:MARG:AREA{Area}:POS:AVER?", "Access"=enum."Read Only", "Range Table"="", "Read Callback"="", "Write Callback"="", "Range Callback"="", "Check Callback"="", "Rngtable Callback"="", "Coerce Callback"="", "Supported Models"="", "Instrument Options"="", "Check Status Callback"="", "Flags"=0, "Help"="Returns spectrum emission mask margin positions for all measured list mode segments.\n\nAvailable Repeated Capabilities:\ninstance: i0, i1, i2, i3, i4, i5, i6, i7, i8, i9, i10, i11, i12, i13, i14, i15, i16, i17, i18, i19, i20, i21, i22, i23, i24, i25, i26, i27, i28, i29, i30, i31, i32\r\nArea: a1, a2, a3, a4, a5, a6, a7, a8, a9, a10, a11, a12\r\n\nRemote-control command(s):\nFETCh:NRMMw:MEAS<i>:MEValuation:LIST:SEMask:MARGin:AREA<no>:POSitiv:AVERage?"}, {"Level"=6, "Class Only"=FALSE, "Identifier"="RSCMXPNRFR2M_ATTR_FETCH_MULTI_EVAL_MEASUREMENT_LIST_SEM_MARGIN_AREA_POSITIVE_CURRENT_RESULTS", "Descriptive Name"="Fetch Multi Eval Measurement List SEM Margin Area Positive Current Results", "Data Type"=enum."RawString", "Command"="FETC:NRMM:MEAS{instance}:MEV:LIST:SEM:MARG:AREA{Area}:POS:CURR?", "Access"=enum."Read Only", "Range Table"="", "Read Callback"="", "Write Callback"="", "Range Callback"="", "Check Callback"="", "Rngtable Callback"="", "Coerce Callback"="", "Supported Models"="", "Instrument Options"="", "Check Status Callback"="", "Flags"=0, "Help"="Returns spectrum emission mask margin positions for all measured list mode segments.\n\nAvailable Repeated Capabilities:\ninstance: i0, i1, i2, i3, i4, i5, i6, i7, i8, i9, i10, i11, i12, i13, i14, i15, i16, i17, i18, i19, i20, i21, i22, i23, i24, i25, i26, i27, i28, i29, i30, i31, i32\r\nArea: a1, a2, a3, a4, a5, a6, a7, a8, a9, a10, a11, a12\r\n\nRemote-control command(s):\nFETCh:NRMMw:MEAS<i>:MEValuation:LIST:SEMask:MARGin:AREA<no>:POSitiv:CURRent?"}, {"Level"=6, "Class Only"=FALSE, "Identifier"="RSCMXPNRFR2M_ATTR_FETCH_MULTI_EVAL_MEASUREMENT_LIST_SEM_MARGIN_AREA_POSITIVE_MINIMUM_RESULTS", "Descriptive Name"="Fetch Multi Eval Measurement List SEM Margin Area Positive Minimum Results", "Data Type"=enum."RawString", "Command"="FETC:NRMM:MEAS{instance}:MEV:LIST:SEM:MARG:AREA{Area}:POS:MIN?", "Access"=enum."Read Only", "Range Table"="", "Read Callback"="", "Write Callback"="", "Range Callback"="", "Check Callback"="", "Rngtable Callback"="", "Coerce Callback"="", "Supported Models"="", "Instrument Options"="", "Check Status Callback"="", "Flags"=0, "Help"="Returns spectrum emission mask margin positions for all measured list mode segments.\n\nAvailable Repeated Capabilities:\ninstance: i0, i1, i2, i3, i4, i5, i6, i7, i8, i9, i10, i11, i12, i13, i14, i15, i16, i17, i18, i19, i20, i21, i22, i23, i24, i25, i26, i27, i28, i29, i30, i31, i32\r\nArea: a1, a2, a3, a4, a5, a6, a7, a8, a9, a10, a11, a12\r\n\nRemote-control command(s):\nFETCh:NRMMw:MEAS<i>:MEValuation:LIST:SEMask:MARGin:AREA<no>:POSitiv:MINimum?"}, {"Level"=4, "Class Only"=TRUE, "Identifier"="", "Descriptive Name"="Segment", "Data Type"=enum."ViInt32", "Command"="", "Access"=enum."Read Only", "Range Table"="", "Read Callback"="", "Write Callback"="", "Range Callback"="", "Check Callback"="", "Rngtable Callback"="", "Coerce Callback"="", "Supported Models"="", "Instrument Options"="", "Check Status Callback"="", "Flags"=0, "Help"="The class for segment in list mode"}, {"Level"=5, "Class Only"=TRUE, "Identifier"="", "Descriptive Name"="ACLR Spectrum", "Data Type"=enum."ViInt32", "Command"="", "Access"=enum."Read Only", "Range Table"="", "Read Callback"="", "Write Callback"="", "Range Callback"="", "Check Callback"="", "Rngtable Callback"="", "Coerce Callback"="", "Supported Models"="", "Instrument Options"="", "Check Status Callback"="", "Flags"=0, "Help"="The following attributes return the ACLR spectrum results for segment in list mode."}, {"Level"=6, "Class Only"=FALSE, "Identifier"="RSCMXPNRFR2M_ATTR_FETCH_MULTI_EVAL_MEASUREMENT_LIST_SEGMENT_ACLR_AVERAGE_RESULTS", "Descriptive Name"="Fetch Multi Eval Measurement List Segment ACLR Average Results", "Data Type"=enum."RawString", "Command"="FETC:NRMM:MEAS{instance}:MEV:LIST:SEGM{Segment}:ACLR:AVER?", "Access"=enum."Read Only", "Range Table"="", "Read Callback"="", "Write Callback"="", "Range Callback"="", "Check Callback"="", "Rngtable Callback"="", "Coerce Callback"="", "Supported Models"="", "Instrument Options"="", "Check Status Callback"="", "Flags"=0, "Help"="Returns ACLR single value results for segment <no> in list mode.\n\nAvailable Repeated Capabilities:\ninstance: i0, i1, i2, i3, i4, i5, i6, i7, i8, i9, i10, i11, i12, i13, i14, i15, i16, i17, i18, i19, i20, i21, i22, i23, i24, i25, i26, i27, i28, i29, i30, i31, i32\r\nSegment: s1, s2, s3, s4, s5, s6, s7, s8, s9, s10, s11, s12, s13, s14, s15, s16, s17, s18, s19, s20, s21, s22, s23, s24, s25, s26, s27, s28, s29, s30, s31, s32, s33, s34, s35, s36, s37, s38, s39, s40, s41, s42, s43, s44, s45, s46, s47, s48, s49, s50, s51, s52, s53, s54, s55, s56, s57, s58, s59, s60, s61, s62, s63, s64, s65, s66, s67, s68, s69, s70, s71, s72, s73, s74, s75, s76, s77, s78, s79, s80, s81, s82, s83, s84, s85, s86, s87, s88, s89, s90, s91, s92, s93, s94, s95, s96, s97, s98, s99, s100, s101, s102, s103, s104, s105, s106, s107, s108, s109, s110, s111, s112, s113, s114, s115, s116, s117, s118, s119, s120, s121, s122, s123, s124, s125, s126, s127, s128, s129, s130, s131, s132, s133, s134, s135, s136, s137, s138, s139, s140, s141, s142, s143, s144, s145, s146, s147, s148, s149, s150, s151, s152, 
